vi "fault_builder.vi"(8 "Fault type":string="BCG", 9 "Event type":string="CL", 10 "Fault time":string="0.023560", 11 "Node fault":dbl) -> (3 "Result":string)   [LabVIEW 2020]
panel:
  # "FAULT BUILDER"
  # "Nó virtual"
  # "nó virtual 2"
  # "SW_source"
  # "SW_load"
  # "Rs"
  # "Rl"
  # "N000VAS000NA       -1.       10.                                             0\n  N000VBS000NB       -1.       10.                                             0\n  N000VCS000NC       -1.       10.                                             0\n  S000NAN0025A       -1.       10.                                             0\n  S000NBN0025B       -1.       10.                                             0\n  S000NCN0025C       -1.       10.                                             0\n  S000NAS000ZA  0.125000       10.                                             0\n  S000NBS000ZB  0.125000       10.                                             0\n  S000NCS000ZC  0.125000       10.                                             0\n  S000GAN000GA  0.125000       10.                                             0\n  S000GBN000GB  0.125000       10.                                             0\n  S000GCN000GC  0.125000       10.                                             0"
  # "nó vitual para encaixar\na estrutura de chaves"
  # "S00Z1A\nS00Z1B\nS00Z1C"
  # "S00Z2A\nS00Z2B\nS00Z2C"
  # "N00__A\nN00__B\nN00__C"
  # "N000VA\nN000VB\nN000VC"
  # "S00Z1A\nS00Z1B\nS00Z1C"
  # "S000NA\nS000NB\nS000NC"
  # "S000NA\nS000NB\nS000NC"
  # "S00Z2A\nS00Z2B\nS00Z2C"
  # "nó do sistema\n(local de falta)"
  # "S000NA\nS000NB\nS000NC"
  # "S000ZA\nS000ZB\nS000ZC"
  # "SW_fault"
  # "S000ZA\nS000ZB\nS000ZC"
  # "S000PA\nS000PB\nS000PC"
  # "RLC"
  # "S000GA\nS000GB\nS000GC"
  # "S00Z3A\nS00Z3B\nS00Z3C"
  # "S000ZAS000GA            100.00                                               0\n  S000ZBS000GB            100.00                                               0\n  S000ZCS000GC            100.00                                               0\n  N000GA                   .0001                                               0\n  N000GB                   .0001                                               0\n  N000GC                   .0001                                               0"
  # "S00Z3A\nS00Z3B\nS00Z3C"
  # "SW_fault_G"
  # "S00Z3G"
  # "S00Z4G"
  # "-> curto"
  # "Rg"
  # "S00Z4G"
  # "Ground"
  # "S000PA\nS000PB\nS000PC"
  # "S000PA\nS000PC\nS000PA"
  # "SW_fault_phases"
  # "S000ZG"
  # "S00Z3G"
  # "Rz"
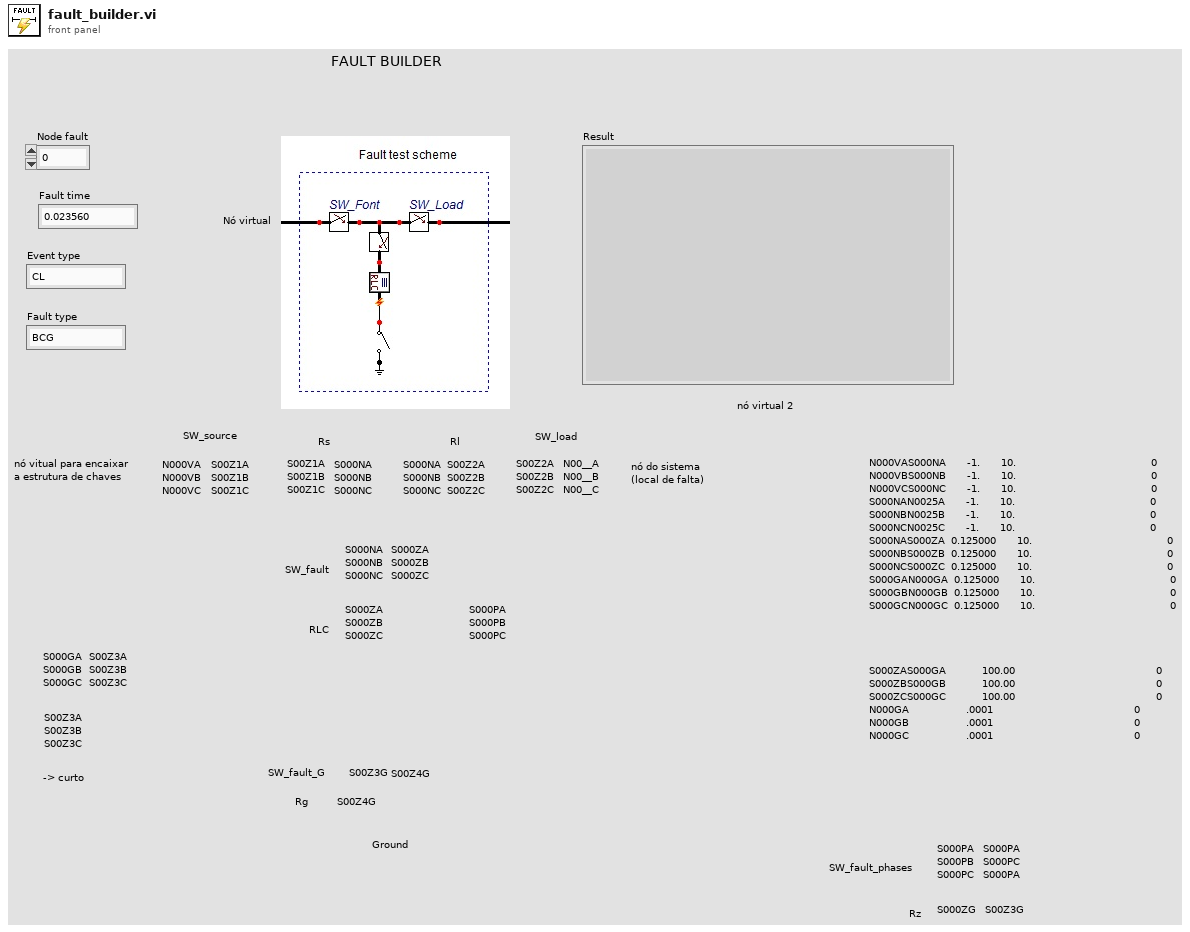
[diagram p1: front panel]
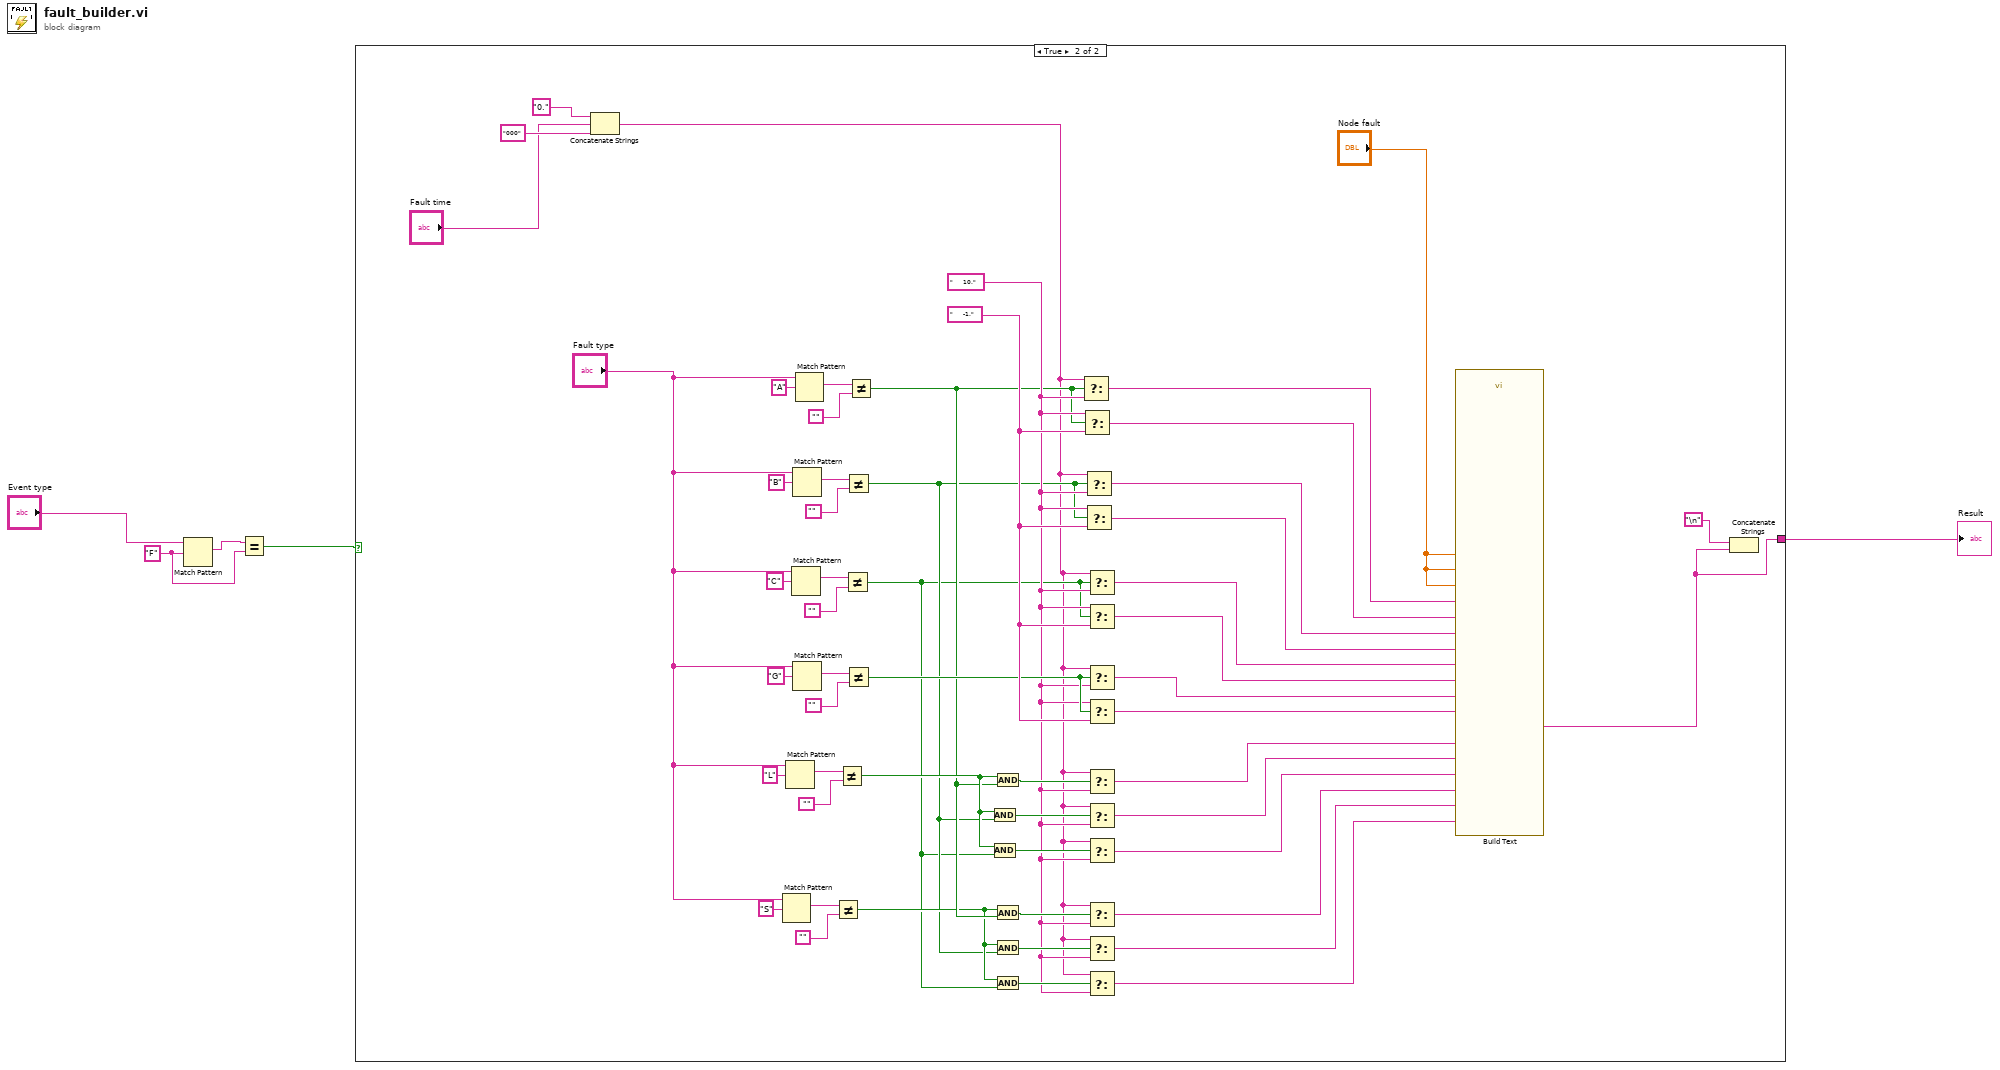
[diagram p0: block diagram]
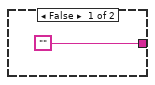
[diagram p2: hidden frame]
diagram:
  w4 = "F" ("regular expression")
  n1 = Match Pattern(string="Event type", regular expression=w4) -> (match substring=w3:string)  [unwired: 1 in, 3 out]
  n2 = Equal?(x=w3, y=w4) -> (x = y?=w2:bool)
  n3 = case shown="True" w2 {
    tunnel: ["" w7] -> w1
    frame False {
    }
    frame True {
      w36 = "     -1."
      w21 = "     10."
      n4 = Concatenate Strings("0." ("string"), "Fault time", "000" ("string")) -> (w9:string)
      n5 = Match Pattern(string="Fault type", regular expression="S") -> (match substring=w44:string)  [unwired: 1 in, 3 out]
      n6 = Match Pattern(string="Fault type", regular expression="L") -> (match substring=w47:string)  [unwired: 1 in, 3 out]
      n7 = Match Pattern(string="Fault type", regular expression="C") -> (match substring=w53:string)  [unwired: 1 in, 3 out]
      n8 = Match Pattern(string="Fault type", regular expression="B") -> (match substring=w56:string)  [unwired: 1 in, 3 out]
      n9 = Match Pattern(string="Fault type", regular expression="G") -> (match substring=w50:string)  [unwired: 1 in, 3 out]
      n10 = Match Pattern(string="Fault type", regular expression="A") -> (match substring=w59:string)  [unwired: 1 in, 3 out]
      n11 = Not Equal?(x=w44, y="") -> (x != y?=w19:bool)
      n12 = Not Equal?(x=w47, y="") -> (x != y?=w28:bool)
      n13 = Not Equal?(x=w53, y="") -> (x != y?=w17:bool)
      n14 = Not Equal?(x=w56, y="") -> (x != y?=w18:bool)
      n15 = Not Equal?(x=w50, y="") -> (x != y?=w35:bool)
      n16 = Not Equal?(x=w59, y="") -> (x != y?=w20:bool)
      n17 = And(x=w28, y=w18) -> (x .and. y?=w30:bool)
      n18 = And(x=w28, y=w17) -> (x .and. y?=w29:bool)
      n19 = And(x=w28, y=w20) -> (x .and. y?=w31:bool)
      n20 = And(x=w19, y=w20) -> (x .and. y?=w24:bool)
      n21 = And(x=w19, y=w18) -> (x .and. y?=w23:bool)
      n22 = And(x=w19, y=w17) -> (x .and. y?=w22:bool)
      n23 = Select(t=w9, s=w20, f=w21) -> (s? t:f=w42:string)
      n24 = Select(t=w21, s=w20, f=w36) -> (s? t:f=w41:string)
      n25 = Select(t=w9, s=w18, f=w21) -> (s? t:f=w40:string)
      n26 = Select(t=w21, s=w18, f=w36) -> (s? t:f=w38:string)
      n27 = Select(t=w9, s=w17, f=w21) -> (s? t:f=w39:string)
      n28 = Select(t=w21, s=w17, f=w36) -> (s? t:f=w37:string)
      n29 = Select(t=w9, s=w35, f=w21) -> (s? t:f=w34:string)
      n30 = Select(t=w21, s=w35, f=w36) -> (s? t:f=w33:string)
      n31 = Select(t=w9, s=w31, f=w21) -> (s? t:f=w27:string)
      n32 = Select(t=w9, s=w30, f=w21) -> (s? t:f=w26:string)
      n33 = Select(t=w9, s=w29, f=w21) -> (s? t:f=w25:string)
      n34 = Select(t=w9, s=w24, f=w21) -> (s? t:f=w16:string)
      n35 = Select(t=w9, s=w23, f=w21) -> (s? t:f=w15:string)
      n36 = Select(t=w9, s=w22, f=w21) -> (s? t:f=w14:string)
      n37 = call "Build Text"("time_open_Af"=w27, "time_open_Bf"=w26, "time_open_Cf"=w25, "outA"="Node fault", "time_open_Ac"=w16, "outB"="Node fault", "time_open_Bc"=w15, "outC"="Node fault", "time_open_Cc"=w14, "time_close_A"=w42, "time_open_A"=w41, "time_close_B"=w40, "time_open_B"=w38, "time_close_C"=w39, "time_open_C"=w37, "time_close_G"=w34, "time_open_G"=w33) -> ("Result"=w7:string)  [unwired: 9 in, 1 out]
      n38 = Concatenate Strings("\n", w7) -> ()  [unwired: 1 out]
    }
  }
  "Result" <- w1
